vi "Find Network Systems.vi"(8 "Error IN":errorcluster caption="error in (no error)") -> (0 "Error OUT":errorcluster caption="error in (no error)", 3 "Serial Number":u32)   [LabVIEW 2019]
uses:
  <vilib>/nisyscfg/nisyscfg.lvlib
  <vilib>/nisyscfg/Close (System).vi
  <resource>/objmgr/nicontrollersysapi.rc
  <vilib>/nisyscfg/Find Hardware.vi
  Type Defs and Controls/TCP Data Stream Mode.ctl
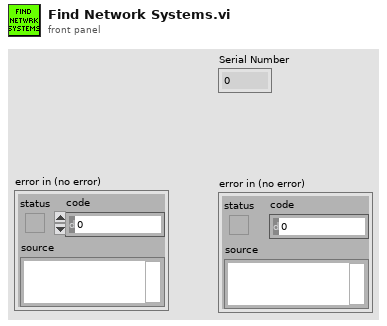
[diagram p1: front panel]
types:
  T1 = typedef "TCP Data Stream Mode.ctl" = enum16{"Init RT", "Init PC", "Connect RT", "Connect PC", "Write Data", "Read Data", "Close"}
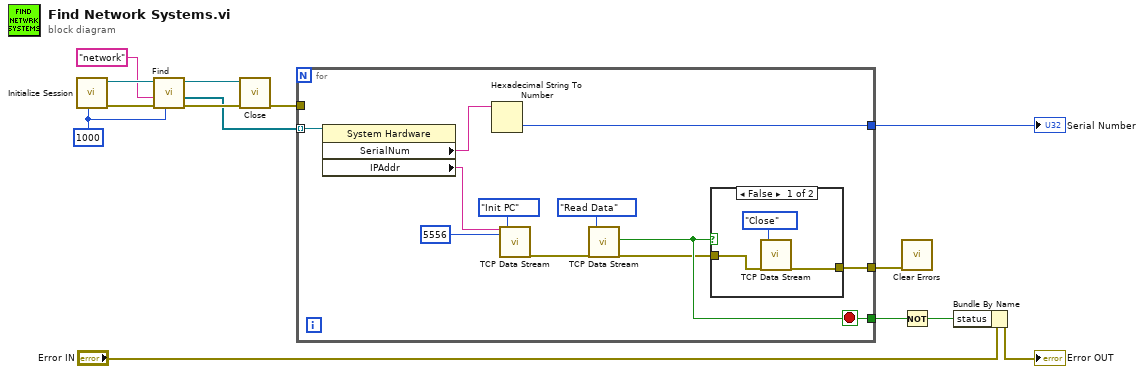
[diagram p0: block diagram]
diagram:
  w8 = u32 1000 ("connect timeout in ms (4s)")
  n1 = call <vilib>:"Initialize Session.vi"("Connect Timeout (4000 ms)"=w8) -> ("error out"=w9:errorcluster, "Session out"=w14:refnum<k21>)  [unwired: 9 in]
  n2 = call-poly <vilib>:"Find.vi"("Remote Timeout (300,000 ms)"=w8, "error in (no error)"=w9, "Experts"="network" ("experts"), "Session in"=w14) -> ("error out"=w12:errorcluster, "Resources out"=w10:refnum<k20>[], "Session out"=w13:refnum<k21>)  [unwired: 4 in, 1 out]
  n3 = call-poly <vilib>:"Close.vi"("error in (no error)"=w12, "Session in"=w13) -> ("error out"=w7:errorcluster)  [unwired: 9 in]
  n4 = for {
    tunnel: w10 -> [w25] mode=indexing
    tunnel: w7 -> [_]
    tunnel: [w23] -> w6
    tunnel: [w17] -> w3
    tunnel: [w15] -> w1
    stop <- w17 stop-if-true
    n5 = property class="System Hardware"(reference=w25) -> ("SerialNum"=w24:string, "IPAddr"=w21:string)  [unwired: 1 in, 2 out]
    n6 = Hexadecimal String To Number(string=w24) -> (number=w23:u32)  [unwired: 2 in, 1 out]
    n7 = call "TCP Data Stream.vi"("Address"=w21, "Port"=u16 5556, "Mode"=TCP_Data_Stream_Mode."Init PC") -> ("Error OUT"=w19:errorcluster)  [unwired: 12 in, 4 out]
    n8 = call "TCP Data Stream.vi"("Error IN"=w19, "Mode"=TCP_Data_Stream_Mode."Read Data") -> ("Connected?"=w17:bool, "Error OUT"=w16:errorcluster)  [unwired: 13 in, 3 out]
    n9 = case shown="False" w17 {
      tunnel: w16 -> [w27 w29]
      tunnel: [w26 w29] -> w15
      frame False {
        n10 = call "TCP Data Stream.vi"("Error IN"=w27, "Mode"=TCP_Data_Stream_Mode."Close") -> ("Error OUT"=w26:errorcluster)  [unwired: 13 in, 4 out]
      }
      frame True {
      }
    }
  }
  "Serial Number" <- w6
  n11 = call <vilib>:"Clear Errors.vi"("error in (no error)"=w1) -> ()  [unwired: 5 in, 2 out]
  n12 = Not(x=w3) -> (.not. x?=w2:bool)
  n13 = Bundle By Name(cluster="Error IN", "status"=w2) -> (→"Error OUT":errorcluster)
